vi "Tracer_CheckEnable.vi"(6 "Calltree Level":i32, 9 "Category":string) -> (1 "Trace Enabled":bool)   [LabVIEW 2018, in "TracerLibrary.lvlib" / "Tracer.lvclass"]
uses:
  Tracer.lvclass
  protected/Tracer_ClassAttributes.vi
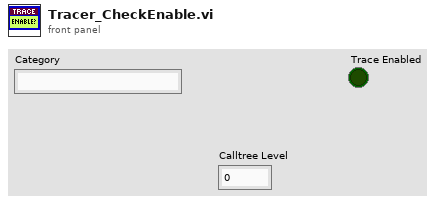
[diagram p1: front panel]
types:
  T1 = typedef "TRACE.lvlib/TRACE.lvclass/TRACE_ObjectAttributes.ctl" = cluster{"TraceContainer":variant}
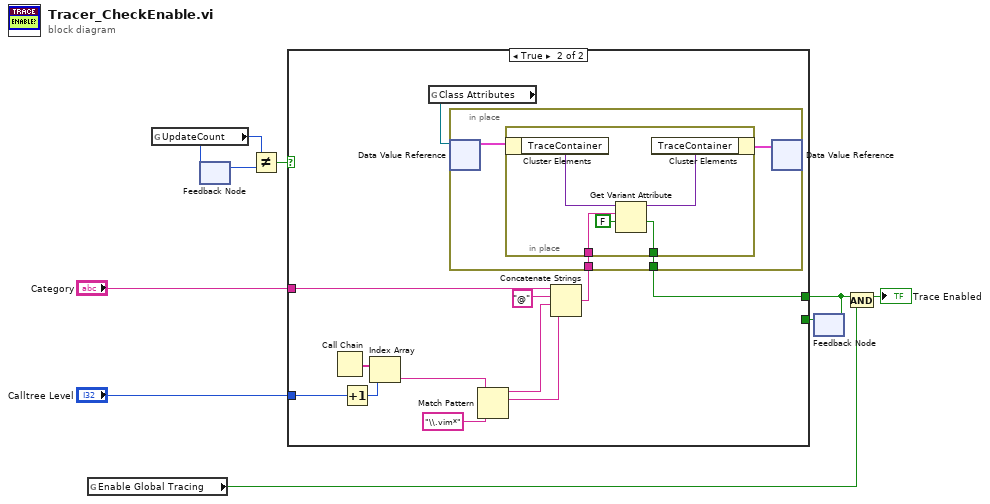
[diagram p0: block diagram]
diagram:
  n1 = global read "Tracer_ClassAttributes.vi" "Enable Global Tracing"() -> (w1:bool)
  n2 = global read "Tracer_ClassAttributes.vi" "UpdateCount"() -> (w5:i32)
  n3 = feedback #1() -> (w6:i32)  [unwired: 1 in]
  n4 = feedback-in #1(w5) -> ()
  n5 = Not Equal?(x=w5, y=w6) -> (x != y?=w7:bool)
  n6 = feedback #2() -> (w4:bool)  [unwired: 1 in]
  n7 = case shown="True" w7 {
    tunnel: "Category" -> [_ w20]
    tunnel: [w10 w16] -> w8
    tunnel: w4 -> [w10 _]
    tunnel: "Calltree Level" -> [_ w12]
    frame False {
    }
    frame True {
      n8 = Call Chain() -> (call chain=w21:string[])
      n9 = Increment(x=w12) -> (x+1=w13:i32)
      n10 = Index Array(array=w21, index=w13) -> (element=w14:string)
      n11 = global read "Tracer_ClassAttributes.vi" "Class Attributes"() -> (w22:refnum<data-value>)
      n12 = Match Pattern(string=w14, regular expression="\\.vim*") -> (before substring=w18:string, match substring=w15:string)  [unwired: 1 in, 2 out]
      n13 = Concatenate Strings(w20, "@" ("string"), w18, w15) -> (w11:string)
      n14 = in-place {
        in-place-border: w11 -> [w26]
        in-place-border: [w25] -> w16
        n15 = in-place-dvr #3(w22) -> (w24:T1)  [unwired: 1 out]
        n16 = in-place {
          in-place-border: w26 -> [w30]
          in-place-border: [w29] -> w25
          n17 = in-place-cluster #4(w24) -> ("TraceContainer"=w28:variant)
          n18 = Get Variant Attribute(Variant=w28, name=w30, default value (empty Variant)=FALSE) -> (duplicate Variant=w27:variant, value=w29:bool)  [unwired: 1 in, 2 out]
          n19 = in-place-cluster #4("TraceContainer"=w27) -> (w23:T1)
        }
        n20 = in-place-dvr #3(w23) -> ()  [unwired: 2 out]
      }
    }
  }
  n21 = feedback-in #2(w8) -> ()
  n22 = And(x=w8, y=w1) -> (x .and. y?=→"Trace Enabled":bool)
